vi "Write.vi"(0 "System Interface":refnum<class "System Interface.lvclass">, 1 "Terminal":string="Output", 5 "Process Data":T1, 11 "Error In":errorcluster) -> (4 "System Interface out":refnum<class "System Interface.lvclass">, 15 "Error Out":errorcluster)   [LabVIEW 2020, in "Optitrack.lvlib"]
uses:
  <vilib>/ADAS Record/CustomDataTypes/Optitrack/Optitrack.lvlib
  414300ae-2f3d-445e-aeca-488e23f625b8.vi
  <vilib>/FlexLogger/SDK/PluginSDK.lvlibp/PEFClasses/SDK/System Interface/System Interface.lvclass
  <vilib>/ADAS Record/CustomDataTypes/Optitrack/Process Data.ctl
  Projects/NI AzDO/Mercedes-MPIC-201077/Record_MPIC3/mercedes-record-mpic3-201077/software-record-plugins/labview-2020/src/shared/TypeDef-Optitrack-RigidBody.ctl
  Projects/NI AzDO/Mercedes-MPIC-201077/Record_MPIC3/mercedes-record-mpic3-201077/software-record-plugins/labview-2020/src/shared/TypeDef-Optitrack-MarkerPoint.ctl
  Projects/NI AzDO/Mercedes-MPIC-201077/Record_MPIC3/mercedes-record-mpic3-201077/software-record-plugins/labview-2020/src/shared/TypeDef-Optitrack-MarkerSet.ctl
  Projects/NI AzDO/Mercedes-MPIC-201077/Record_MPIC3/mercedes-record-mpic3-201077/software-record-plugins/labview-2020/src/shared/TypeDef-Optitrack-LabeledMarker.ctl
  Projects/NI AzDO/Mercedes-MPIC-201077/Record_MPIC3/mercedes-record-mpic3-201077/software-record-plugins/labview-2020/src/shared/TypeDef-Optitrack-TrackedData.ctl
  Projects/NI AzDO/Mercedes-MPIC-201077/Record_MPIC3/mercedes-record-mpic3-201077/software-record-plugins/labview-2020/src/shared/TypeDef-Optitrack-FrameData.ctl
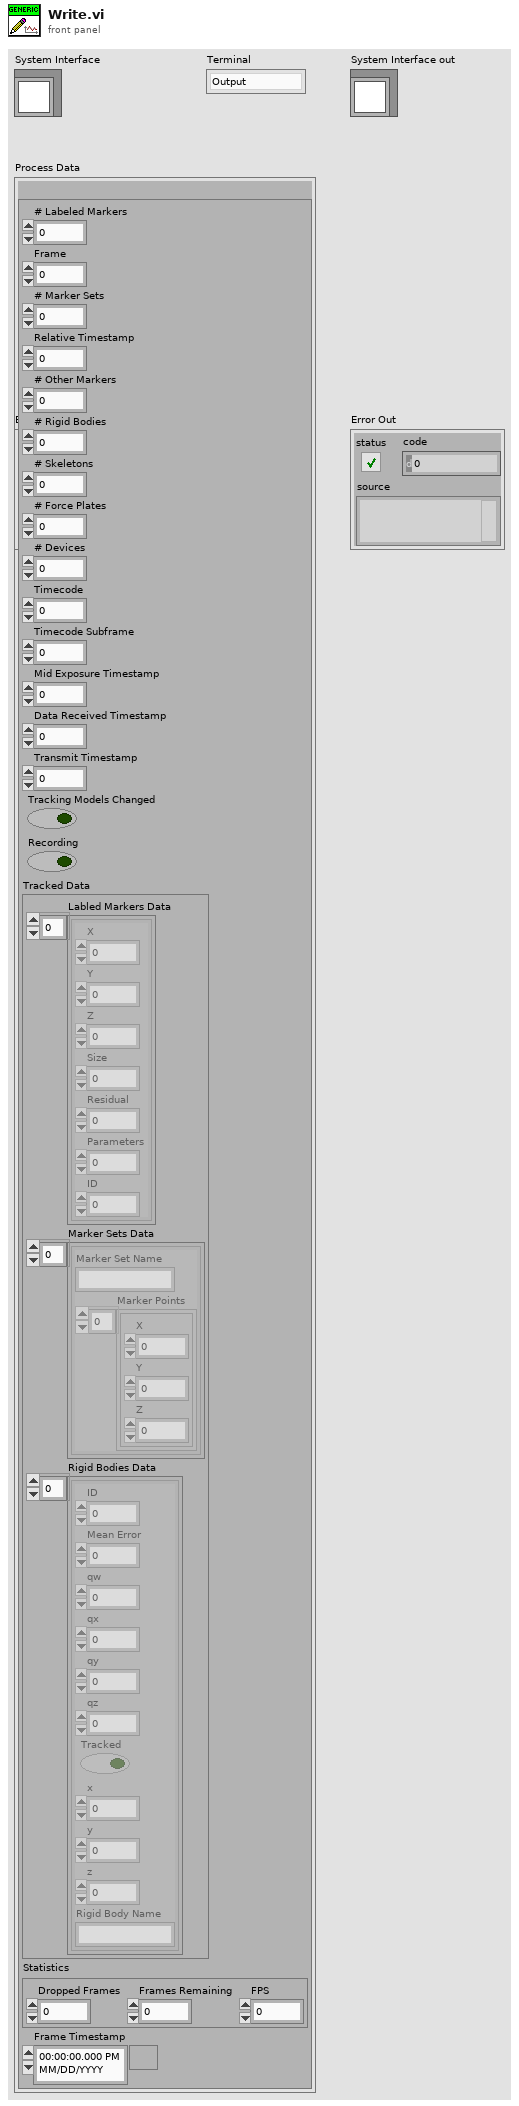
[diagram p1: front panel]
types:
  T1 = typedef "Optitrack.lvlib/Process Data.ctl" = cluster{"OptitrackFrame":T2}
  T2 = typedef "TypeDef-Optitrack-FrameData.ctl" = cluster{"# Labeled Markers":i32, "Frame":i32, "# Marker Sets":i32, "Relative Timestamp":dbl, "# Other Markers":i32, "# Rigid Bodies":i32, "# Skeletons":i32, "# Force Plates":i32, "# Devices":i32, "Timecode":u32, "Timecode Subframe":u32, "Mid Exposure Timestamp":u64, "Data Received Timestamp":u64, "Transmit Timestamp":u64, "Tracking Models Changed":bool, "Recording":bool, "Tracked Data":T3, "Statistics":cluster{"Dropped Frames":i32, "Frames Remaining":i32, "FPS":dbl}, "Frame Timestamp":timestamp}
  T3 = typedef "TypeDef-Optitrack-TrackedData.ctl" = cluster{"Labled Markers Data":T4[], "Marker Sets Data":T5[], "Rigid Bodies Data":T7[]}
  T4 = typedef "TypeDef-Optitrack-LabeledMarker.ctl" = cluster{"X":sgl, "Y":sgl, "Z":sgl, "Size":sgl, "Residual":sgl, "Parameters":i16, "ID":i32}
  T5 = typedef "TypeDef-Optitrack-MarkerSet.ctl" = cluster{"Marker Set Name":string, "Marker Points":T6[]}
  T6 = typedef "TypeDef-Optitrack-MarkerPoint.ctl" = cluster{"X":sgl, "Y":sgl, "Z":sgl}
  T7 = typedef "TypeDef-Optitrack-RigidBody.ctl" = cluster{"ID":i32, "Mean Error":sgl, "qw":sgl, "qx":sgl, "qy":sgl, "qz":sgl, "Tracked":bool, "x":sgl, "y":sgl, "z":sgl, "Rigid Body Name":string}
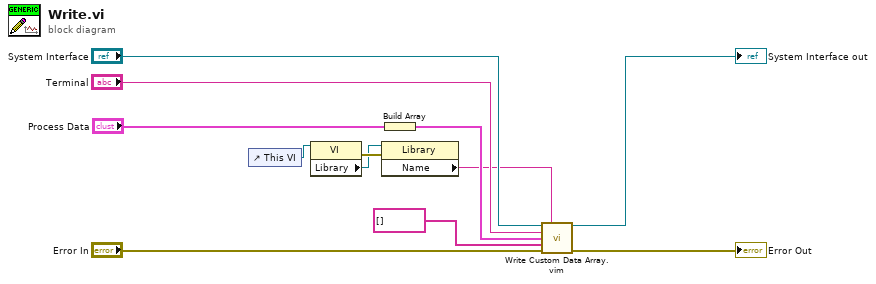
[diagram p0: block diagram]
diagram:
  n1 = control-ref of="This VI"() -> (w5:refnum<vi>)
  n2 = property class="VI"(reference=w5) -> (error out=w4:errorcluster, "Library"=w3:refnum<vi>)  [unwired: 1 in, 1 out]
  n3 = property class="Library"(reference=w3, error in=w4) -> ("Name"=w2:string)  [unwired: 2 out]
  n4 = Build Array("Process Data") -> (w7:T1[])
  n5 = call "Write Custom Data Array.vim"("System Interface"="System Interface", "Type"=w2, "Terminal"="Terminal", "Data"=w7, "Metadata"=string[] [], "error in (no error)"="Error In") -> ("System Interface out"=→"System Interface out":refnum<class "System Interface.lvclass">, "error out"=→"Error Out":errorcluster)  [unwired: 8 in]
